vi "Constants.vi"() -> ()   [LabVIEW 2017]
panel:
  in  "Transceiver Build Spec Name":string="UDP Transceiver"
  in  "Path to UDP Project":path=path "C:/github/data-sharing-framework/Data Sharing Framework/Source/Transceivers/UDP/UDP Transceiver Build.lvproj"
  in  "Path to Common Dev Directory":path=path "C:/Builds/Data Sharing Framework/Current"
  in  "Windows Install Directories":path[](array[path])=[path "C:/DSF", path "C:/DSF/Distributions/Pharlap"]
  in  "Core Build Spec Name":string="Data Sharing Framework Core"
  in  "Target Names":string[](array[string])=["My Computer", "RT PXI Target"]
  in  "Path to core project":path=path "C:/github/data-sharing-framework/Data Sharing Framework/Source/Core/Data Sharing Framework Core Build.lvproj"
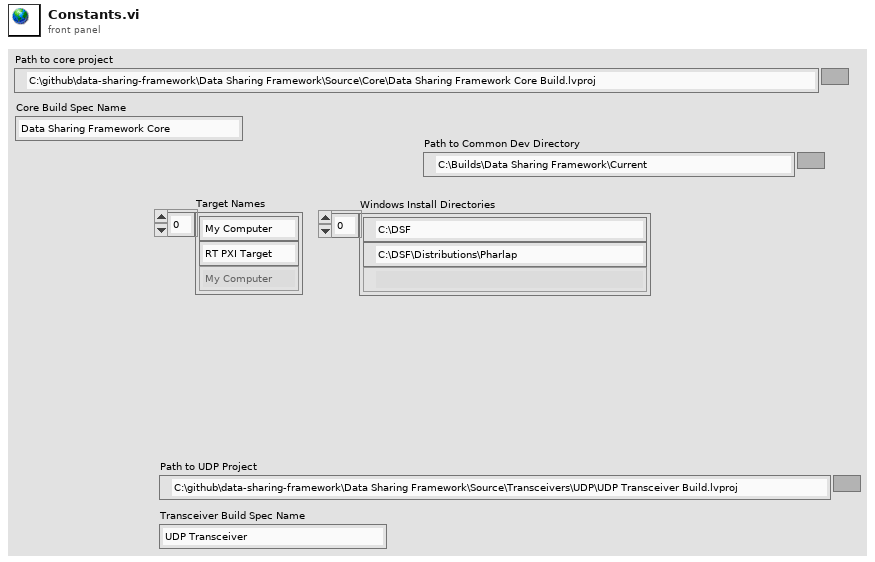
[diagram p1: front panel]
diagram:
